vi "setOutput.vi"(8 "error in (no error)":errorcluster, 10 "output":string, 11 "PrettyPrinting.lvclass in":refnum<class "PrettyPrinting.lvclass">) -> (0 "error out":errorcluster, 3 "PrettyPrinting.lvclass out":refnum<class "PrettyPrinting.lvclass">)   [LabVIEW 2011, in "Views.lvlib" / "ViewerTools.lvlib" / "PrettyPrinting.lvclass"]
uses:
  PrettyPrinting.lvclass
  PrettyPrinting.lvclass/PrettyPrinting.ctl
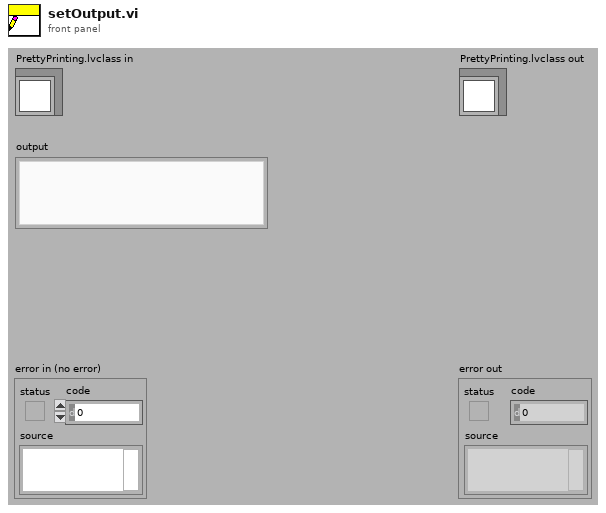
[diagram p1: front panel]
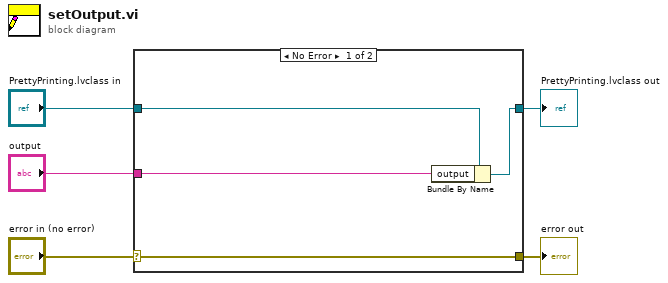
[diagram p0: block diagram]
diagram:
  n1 = case shown="No Error" "error in (no error)" {
    selector: "error in (no error)" -> [w9 w10]
    tunnel: [w9 w10] -> w4
    tunnel: [w7 w11] -> w2
    tunnel: "PrettyPrinting.lvclass in" -> [w8 w11]
    tunnel: "output" -> [w6 _]
    frame No Error {
      n2 = Bundle By Name(cluster=w8, "output"=w6) -> (w7:refnum<class "PrettyPrinting.lvclass">)
    }
    frame Error {
    }
  }
  "error out" <- w4
  "PrettyPrinting.lvclass out" <- w2
